vi "loadDigitalConfig.vi"(8 "error in (no error)":errorcluster, 9 "Channel.lvclass":refnum<class "Channel.lvclass">, 10 "xmlNode.lvclass":refnum<class "xmlNode.lvclass">, 11 "deviceDataBase in":refnum<class "deviceDataBase.lvclass">) -> (0 "error out":errorcluster, 1 "Channel.lvclass out":refnum<class "Channel.lvclass">, 2 "xmlNode out":refnum<class "xmlNode.lvclass">, 3 "deviceDataBase out":refnum<class "deviceDataBase.lvclass">)   [LabVIEW 2009, in "Tools.lvlib" / "DatabaseHelpers.lvlib" / "deviceDataBase.lvclass"]
uses:
  deviceDataBase.lvclass
  xmlNode/xmlNode.lvclass
  Database Objects/Channel/Channel.lvclass
  Database Objects/Channel/DigitalChannel/DigitalChannel.lvclass
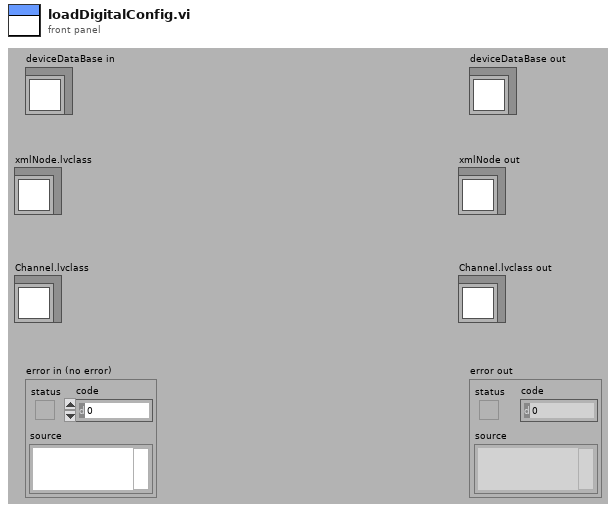
[diagram p1: front panel]
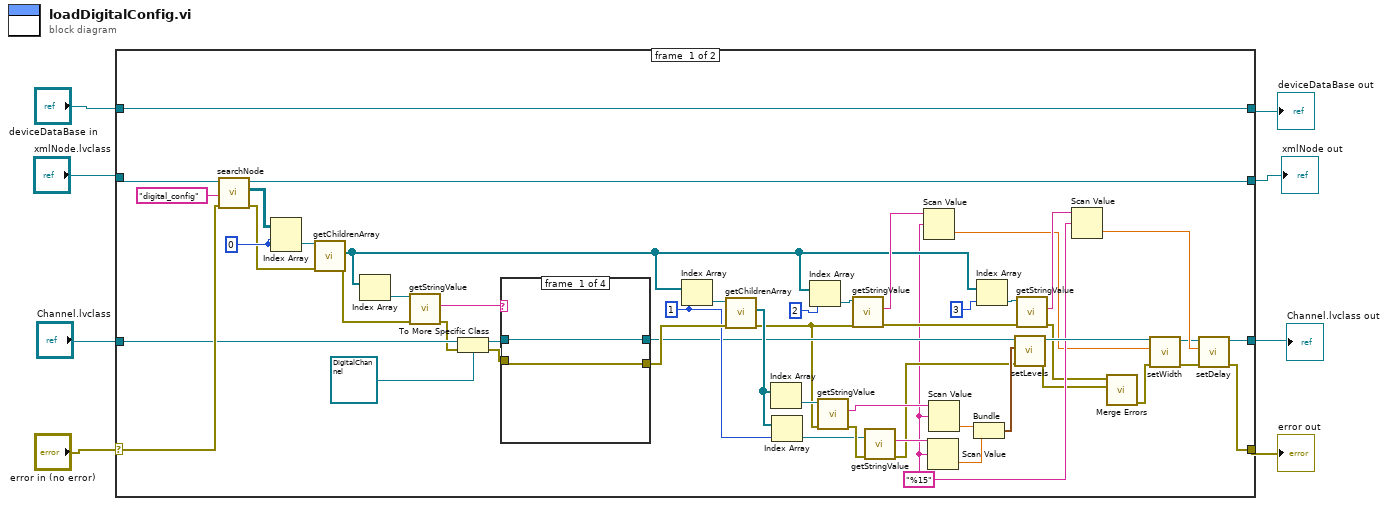
[diagram p0: block diagram]
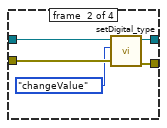
[diagram p2: hidden frame]
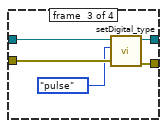
[diagram p3: hidden frame]
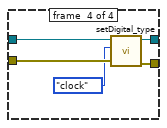
[diagram p4: hidden frame]
diagram:
  n1 = case shown="No Error" "error in (no error)" {
    selector: "error in (no error)" -> [w56 w78]
    tunnel: [w13 w78] -> w7
    tunnel: [w59 w77] -> w5
    tunnel: "deviceDataBase in" -> [w59 w77]
    tunnel: "xmlNode.lvclass" -> [w58 _]
    tunnel: "Channel.lvclass" -> [w48 _]
    tunnel: [w55 _] -> w2
    tunnel: [w11 _] -> w1
    frame #0 {
      w20 = "%15"
      w40 = 1
      w53 = 0
      n2 = call-dynamic "searchNode.vi"("error in (no error)"=w56, "searchElementName"="digital_config", "xmlNode in"=w58) -> ("error out"=w51:errorcluster, "arrayXmlNodes"=w54:refnum<class "xmlNode.lvclass">[][], "xmlNode out"=w55:refnum<class "xmlNode.lvclass">)  [unwired: 6 in]
      n3 = Index Array(array=w54, index (row)=w53, index (col)=w53) -> (element=w52:refnum<class "xmlNode.lvclass">)
      n4 = call-dynamic "getChildrenArray.vi"("error in (no error)"=w51, "xmlNode.lvclass in"=w52) -> ("error out"=w49:errorcluster, "Children"=w24:refnum<class "xmlNode.lvclass">[])  [unwired: 7 in, 1 out]
      n5 = Index Array(array=w24) -> (element=w50:refnum<class "xmlNode.lvclass">)  [unwired: 1 in]
      n6 = call-dynamic "getStringValue.vi"("error in (no error)"=w49, "xmlNode.lvclass in"=w50) -> ("error out"=w46:errorcluster, "stringValue"=w44:string)  [unwired: 7 in, 1 out]
      n7 = To More Specific Class(target class=refnum<class "DigitalChannel.lvclass"> refnum ("Tools.lvlib:DatabaseHelpers.lvlib:DigitalChannel.lvclass"), reference=w48, error in=w46) -> (specific class reference=w47:refnum<class "DigitalChannel.lvclass">, error out=w45:errorcluster)
      n8 = case shown="\"changeValue\"" w44 {
        tunnel: w47 -> [w61 w66 w71 w76]
        tunnel: w45 -> [w60 w65 w70 w75]
        tunnel: [w61 w63 w68 w73] -> w32
        tunnel: [w60 w62 w67 w72] -> w42
        frame #0 {
        }
        frame #1 {
          n9 = call "setDigital_type.vi"("error in (no error)"=w65, "digital_type"=enum16{"changeValue", "pulse", "clock"}."changeValue", "DigitalChannel.lvclass in"=w66) -> ("error out"=w62:errorcluster, "DigitalChannel.lvclass out"=w63:refnum<class "DigitalChannel.lvclass">)  [unwired: 7 in]
        }
        frame #2 {
          n10 = call "setDigital_type.vi"("error in (no error)"=w70, "digital_type"=enum16{"changeValue", "pulse", "clock"}."pulse", "DigitalChannel.lvclass in"=w71) -> ("error out"=w67:errorcluster, "DigitalChannel.lvclass out"=w68:refnum<class "DigitalChannel.lvclass">)  [unwired: 7 in]
        }
        frame #3 {
          n11 = call "setDigital_type.vi"("error in (no error)"=w75, "digital_type"=enum16{"changeValue", "pulse", "clock"}."clock", "DigitalChannel.lvclass in"=w76) -> ("error out"=w72:errorcluster, "DigitalChannel.lvclass out"=w73:refnum<class "DigitalChannel.lvclass">)  [unwired: 7 in]
        }
      }
      n12 = Index Array(array=w24, index=w40) -> (element=w43:refnum<class "xmlNode.lvclass">)
      n13 = call-dynamic "getChildrenArray.vi"("error in (no error)"=w42, "xmlNode.lvclass in"=w43) -> ("error out"=w27:errorcluster, "Children"=w41:refnum<class "xmlNode.lvclass">[])  [unwired: 7 in, 1 out]
      n14 = Index Array(array=w41) -> (element=w39:refnum<class "xmlNode.lvclass">)  [unwired: 1 in]
      n15 = Index Array(array=w41, index=w40) -> (element=w37:refnum<class "xmlNode.lvclass">)
      n16 = Index Array(array=w24, index=2) -> (element=w29:refnum<class "xmlNode.lvclass">)
      n17 = call-dynamic "getStringValue.vi"("error in (no error)"=w27, "xmlNode.lvclass in"=w39) -> ("error out"=w38:errorcluster, "stringValue"=w36:string)  [unwired: 7 in, 1 out]
      n18 = call-dynamic "getStringValue.vi"("error in (no error)"=w27, "xmlNode.lvclass in"=w29) -> ("error out"=w22:errorcluster, "stringValue"=w26:string)  [unwired: 7 in, 1 out]
      n19 = call-dynamic "getStringValue.vi"("error in (no error)"=w38, "xmlNode.lvclass in"=w37) -> ("error out"=w30:errorcluster, "stringValue"=w35:string)  [unwired: 7 in, 1 out]
      n20 = Scan Value(string=w26, format string=w20) -> (value=w18:dbl)  [unwired: 1 in, 1 out]
      n21 = Scan Value(string=w35, format string=w20) -> (value=w33:dbl)  [unwired: 1 in, 1 out]
      n22 = Scan Value(string=w36, format string=w20) -> (value=w34:dbl)  [unwired: 1 in, 1 out]
      n23 = Bundle(w34, w33) -> (w31:cluster{dbl, dbl})  [unwired: 1 in]
      n24 = Index Array(array=w24, index=3) -> (element=w23:refnum<class "xmlNode.lvclass">)
      n25 = call "setLevels.vi"("error in (no error)"=w30, "levels"=w31, "DigitalChannel.lvclass in"=w32) -> ("error out"=w15:errorcluster, "DigitalChannel.lvclass out"=w28:refnum<class "DigitalChannel.lvclass">)  [unwired: 7 in]
      n26 = call-dynamic "getStringValue.vi"("error in (no error)"=w22, "xmlNode.lvclass in"=w23) -> ("error out"=w16:errorcluster, "stringValue"=w21:string)  [unwired: 7 in, 1 out]
      n27 = Scan Value(string=w21, format string=w20) -> (value=w19:dbl)  [unwired: 1 in, 1 out]
      n28 = call <vilib>:"Merge Errors.vi"("error in 2 (no error)"=w15, "error in 1 (no error)"=w16) -> ("error out"=w14:errorcluster)  [unwired: 5 in]
      n29 = call "setWidth.vi"("error in (no error)"=w14, "width"=w18, "DigitalChannel.lvclass in"=w28) -> ("error out"=w17:errorcluster, "DigitalChannel.lvclass out"=w12:refnum<class "DigitalChannel.lvclass">)  [unwired: 7 in]
      n30 = call "setDelay.vi"("error in (no error)"=w17, "delay"=w19, "DigitalChannel.lvclass in"=w12) -> ("error out"=w13:errorcluster, "DigitalChannel.lvclass out"=w11:refnum<class "DigitalChannel.lvclass">)  [unwired: 7 in]
    }
    frame #1 {
    }
  }
  "error out" <- w7
  "deviceDataBase out" <- w5
  "xmlNode out" <- w2
  "Channel.lvclass out" <- w1
